vi "AFT Create FIR LMS.vi"   [LabVIEW 2017, in "NI_AdaptiveFilter.lvlib"]
doc: "Creates a finite impulse response (FIR) adaptive filter with the standard least mean squares (LMS) algorithm. If you specify a nonzero value for the <B>leakage</B> input, this VI creates an FIR adaptive filter with the leaky LMS algorithm. You must manually select the polymorphic instance you want to use."
uses:
  <vilib>/addons/Adaptive Filters/NI_AdaptiveFilter.lvlib
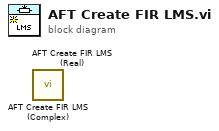
[diagram p0: block diagram]
diagram:
  n1 = call <vilib>:"AFT Create FIR LMS (Complex).vi"() -> ()  [unwired: 10 in, 2 out]
  n2 = call <vilib>:"AFT Create FIR LMS (Real).vi"() -> ()  [unwired: 10 in, 2 out]
